vi "Simple TCP 채팅- Client.vi"() -> ()   [LabVIEW 2018]
doc: "Demonstrates how to open a connection to an TCP server, read the data being sent, and display the data on a chart. This VI is designed to stop if the TCP connection is terminated."
panel:
  in  "보낼 메세지":string
  out "서버에서 받은 문자열":string
  in  "Server Closed":string="The server VI closed the connection."
  in  "Stop":bool
  # "Overview: Demonstrates the use of the TCP functions to connect to a TCP server VI and receive data.\nInstructions:\n1. Ensure Simple TCP - Server.vi is already running.\n2. Run the VI.\n3. Click Stop to stop the VI. Note that if you stop the server VI, this VI will stop automatically."
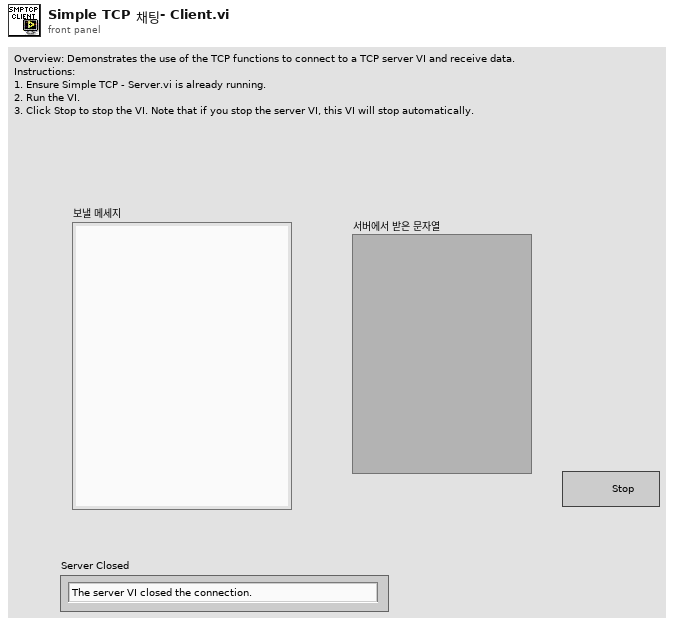
[diagram p1: front panel]
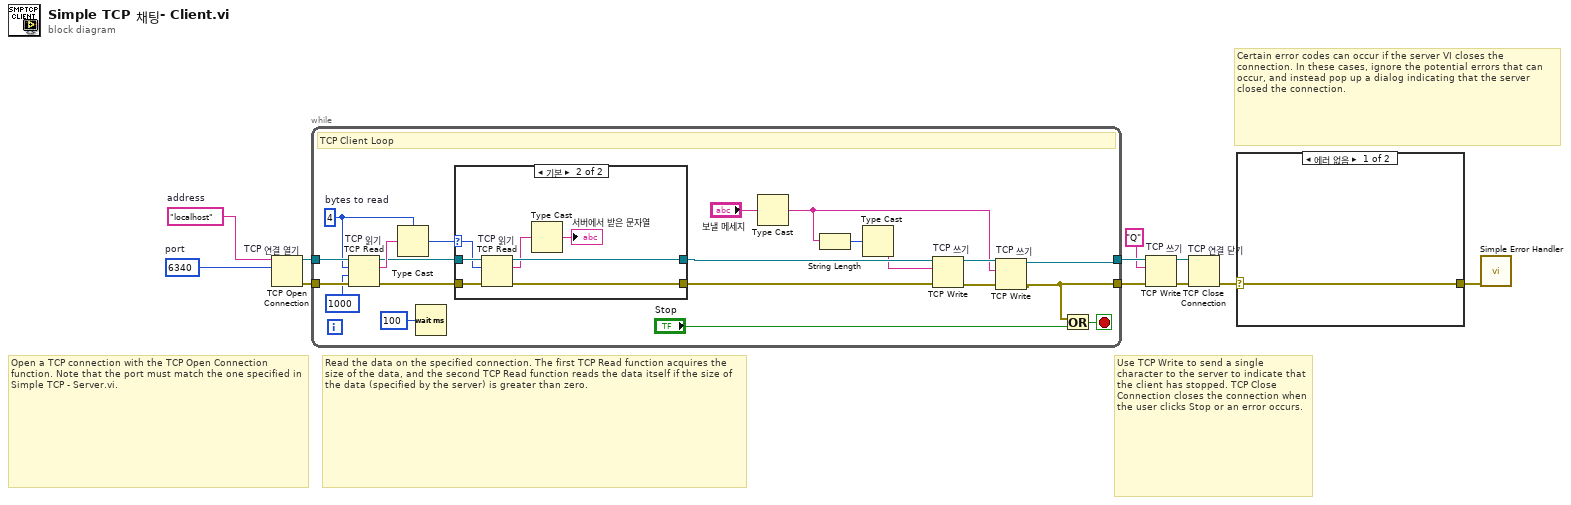
[diagram p0: block diagram]
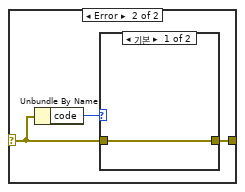
[diagram p2: hidden frame]
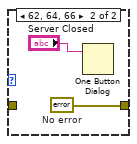
[diagram p3: hidden frame]
diagram:
  w1 = u16 6340  # port
  w2 = "localhost"  # address
  # "Certain error codes can occur if the server VI closes the connection. In these cases, ignore the potential errors that can occur, and instead pop up a dialog indicating that the server closed the connection."
  # "Use TCP Write to send a single character to the server to indicate that the client has stopped. TCP Close Connection closes the connection when the user clicks Stop or an error occurs."
  # "Read the data on the specified connection. The first TCP Read function acquires the size of the data, and the second TCP Read function reads the data itself if the size of the data (specified by the server) is greater than zero."
  # "Open a TCP connection with the TCP Open Connection function. Note that the port must match the one specified in Simple TCP - Server.vi."
  n1 = TCP Open Connection "TCP 연결 열기"(address=w2, remote port or service name=w1) -> (connection ID=w11:refnum<k5>, error out=w10:errorcluster)  [unwired: 3 in]
  n2 = while {
    tunnel: w10 -> [w28]
    tunnel: w11 -> [w29]
    tunnel: [w17] -> w8
    tunnel: [w16] -> w6
    stop <- w25 stop-if-true
    w27 = 4  # bytes to read
    # "TCP Client Loop"
    n3 = TCP Read "TCP 읽기"(connection ID=w29, bytes to read=w27, error in (no error)=w28, 9:1000 ("timeout ms (25000)")) -> (connection ID out=w31:refnum<k5>, data out=w32:string, error out=w30:errorcluster)  [unwired: 1 in]
    n4 = Type Cast(type=w27, x=w32) -> (*(type *) &x=w23:i32)
    n5 = Wait (ms)(milliseconds to wait=u32 100) -> ()  [unwired: 1 out]
    n6 = case shown="기본" w23 {
      selector: w23 -> [_ w36]
      tunnel: w31 -> [w34 w41]
      tunnel: w30 -> [w33 w40]
      tunnel: [w34 w39] -> w21
      tunnel: [w33 w38] -> w20
      frame ..0 {
        # "The server has not written any data"
      }
      frame Default {
        n7 = TCP Read "TCP 읽기"(connection ID=w41, bytes to read=w36, error in (no error)=w40) -> (connection ID out=w39:refnum<k5>, data out=w37:string, error out=w38:errorcluster)  [unwired: 2 in]
        n8 = Type Cast(x=w37) -> (*(type *) &x=→"서버에서 받은 문자열":string)  [unwired: 1 in]
      }
    }
    n9 = Type Cast(x="보낼 메세지") -> (*(type *) &x=w12:string)  [unwired: 1 out]
    n10 = String Length(string=w12) -> (length=w14:i32)
    n11 = Type Cast(x=w14) -> (*(type *) &x=w13:string)  [unwired: 1 out]
    n12 = TCP Write "TCP 쓰기"(connection ID=w21, data in=w13, error in (no error)=w20) -> (connection ID out=w19:refnum<k5>, error out=w18:errorcluster)  [unwired: 2 out]
    n13 = TCP Write "TCP 쓰기"(connection ID=w19, data in=w12, error in (no error)=w18) -> (connection ID out=w17:refnum<k5>, error out=w16:errorcluster)  [unwired: 2 out]
    n14 = Or(x=w16, y="Stop") -> (x .or. y?=w25:bool)
  }
  n15 = TCP Write "TCP 쓰기"(connection ID=w8, data in="Q", error in (no error)=w6) -> (connection ID out=w9:refnum<k5>, error out=w7:errorcluster)  [unwired: 2 out]
  n16 = TCP Close Connection "TCP 연결 닫기"(connection ID=w9, error in (no error)=w7) -> (error out=w4:errorcluster)  [unwired: 1 in, 1 out]
  n17 = case shown="에러 없음" w4 {
    selector: w4 -> [w42 w44]
    tunnel: [w42 w43] -> w3
    frame No Error {
    }
    frame Error {
      n18 = Unbundle By Name(w44) -> ("code"=w45:i32)
      n19 = case shown="기본" w45 {
        tunnel: w44 -> [w46 _]
        tunnel: [w46 w48] -> w43
        frame Default {
        }
        frame 62, 64, 66 {
          w48 = errorcluster {"status"=FALSE, "code"=0, "source"=""}  # No error
          n20 = One Button Dialog(message="Server Closed") -> ()  [unwired: 1 in, 1 out]
        }
      }
    }
  }
  n21 = call <vilib>:"Simple Error Handler.vi"("error in (no error)"=w3) -> ()  [unwired: 4 in, 5 out]
